vi "ComputeUniquePortMap.vi"(9 "port":u32, 10 "board":u32, 11 "PortMap In":u32) -> (3 "PortMap out":u32)   [LabVIEW 2020, in "AIM664LV.lvlib"]
doc: "This function allows you to obtain a portmap based on the portmap value or board/port combination."
uses:
  AIM664LV.lvlib
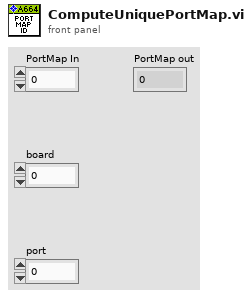
[diagram p1: front panel]
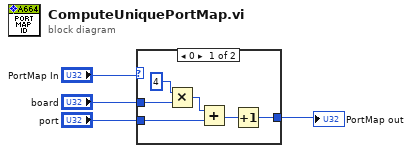
[diagram p0: block diagram]
diagram:
  n1 = case shown="0" "PortMap In" {
    selector: "PortMap In" -> [_ w11]
    tunnel: [w5 w11] -> w1
    tunnel: "board" -> [w7 _]
    tunnel: "port" -> [w6 _]
    frame 0 {
      n2 = Multiply(x=u32 4, y=w7) -> (x*y=w9:u32)
      n3 = Add(x=w9, y=w6) -> (x+y=w8:u32)
      n4 = Increment(x=w8) -> (x+1=w5:u32)
    }
    frame Default {
    }
  }
  "PortMap out" <- w1
